vi "Draw Text on Zone.vi"(7 "[user-specified font]":T1={"Font Name:"="Arial Bold", "Size"=30, "Strikeout?"=FALSE, "Italic?"=FALSE, "Underline?"=FALSE, "Outline?"=FALSE, "Shadow?"=FALSE, "Bold?"=TRUE}, 9 "Name":string, 10 "rect":T2, 11 "Field":picture) -> (3 "new picture":picture)   [LabVIEW 2015]
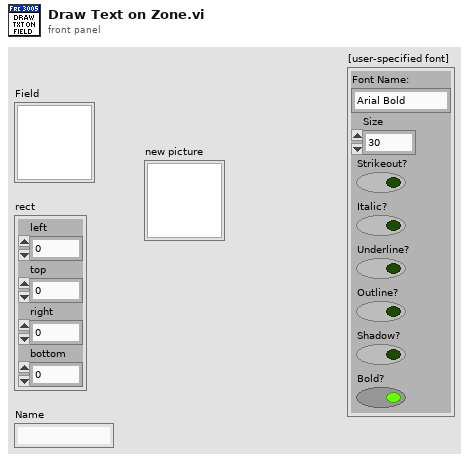
[diagram p1: front panel]
types:
  T1 = cluster{"Font Name:":string, "Size":i16, "Strikeout?":bool, "Italic?":bool, "Underline?":bool, "Outline?":bool, "Shadow?":bool, "Bold?":bool}
  T2 = cluster{"left":i16, "top":i16, "right":i16, "bottom":i16}
  T3 = cluster{"horizontal":enum16{"left", "center", "right"}, "vertical":enum16{"top", "center", "bottom"}}
  T4 = enum16{"User-specified Font", "Application Font", "System Font", "Dialog Font"}
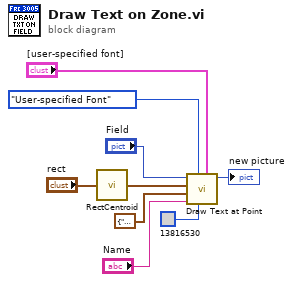
[diagram p0: block diagram]
diagram:
  n1 = call <vilib>:"RectCentroid.vi"("rect"="rect") -> ("point"=w7:cluster{"x":i16, "y":i16})
  n2 = call <vilib>:"Draw Text at Point.vi"("[user-specified font]"="[user-specified font]", "text color(black)"=u32 13816530, "desired font(Application)"=T4."User-specified Font", "text"="Name", "alignment(left, top)"=T3 {"horizontal"=enum."center", "vertical"=enum."center"}, "origin"=w7, "picture"="Field") -> ("new picture"=→"new picture":picture)  [unwired: 3 in, 1 out]
